vi "Set User_Access.vi"(8 "error in (no error)":errorcluster, 9 "Connected Client Cluster":T1, 10 "GUID":string, 11 "Function in":refnum<class "Function.lvclass">) -> (0 "error out":errorcluster, 3 "Function out":refnum<class "Function.lvclass">)   [LabVIEW 2016, in "Function Actor.lvlib" / "Function.lvclass"]
uses:
  <userlib>/Common Components/Function Actor/Function.lvclass
  <userlib>/Common Components/Common/Connected Client Cluster.ctl
  <userlib>/Common Components/Function Actor/Function.lvclass/Function.ctl
  <userlib>/Common Components/Common/Common.lvlib
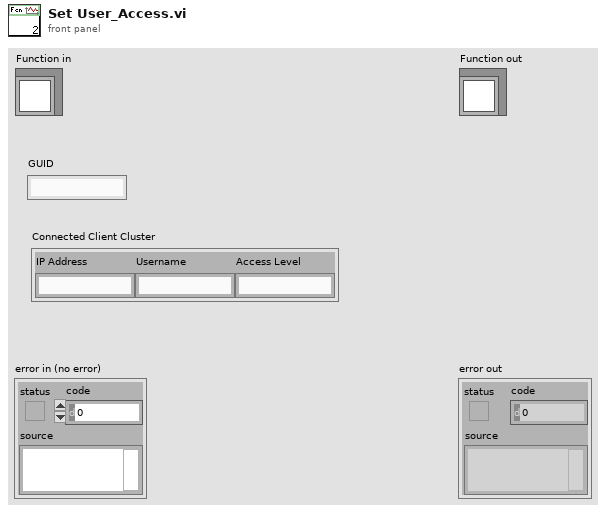
[diagram p1: front panel]
types:
  T1 = typedef "Common.lvlib/Connected Client Cluster.ctl" = cluster{"IP Address":string, "Username":string, "Access Level":string}
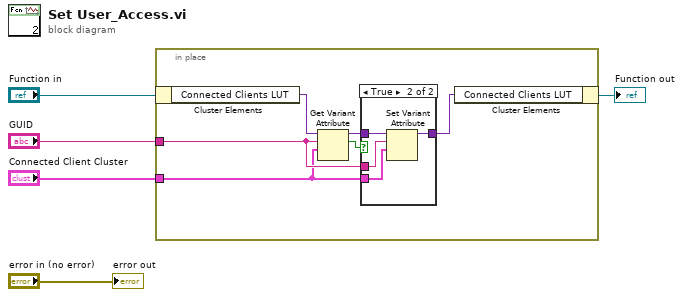
[diagram p0: block diagram]
diagram:
  n1 = in-place {
    in-place-border: "GUID" -> [w8]
    in-place-border: "Connected Client Cluster" -> [w7]
    n2 = in-place-cluster #1("Function in") -> ("Connected Clients LUT"=w11:variant)
    n3 = Get Variant Attribute(Variant=w11, name=w8, default value (empty Variant)=w7) -> (duplicate Variant=w9:variant, found=w10:bool)  [unwired: 1 in, 2 out]
    n4 = case shown="True" w10 {
      tunnel: w9 -> [w12 w16]
      tunnel: w8 -> [_ w15]
      tunnel: w7 -> [_ w14]
      tunnel: [w12 w13] -> w6
      frame False {
      }
      frame True {
        n5 = Set Variant Attribute(Variant=w16, name=w15, value=w14) -> (Variant out=w13:variant)  [unwired: 1 in, 2 out]
      }
    }
    n6 = in-place-cluster #1("Connected Clients LUT"=w6) -> (→"Function out":refnum<class "Function.lvclass">)
  }
  "error out" <- "error in (no error)"
